vi "Set Or Get Selection Area.vi"(8 "error in (no error)":errorcluster caption="错误输入（无错误）", 9 "Mode":T3, 10 "选择区域输入":T1, 11 "Table Ref In":refnum<vi>) -> (0 "error out":errorcluster caption="错误输出", 2 "选择区域输出":T1, 3 "Table Ref Out":refnum<vi>)   [LabVIEW 2012, in "Table Tool.lvlib"]
uses:
  Table Tool.lvlib
  GetOrSet.ctl
  Selection Area.ctl
  <vilib>/Utility/miscctls.llb/LVRowAndColumnTypeDef.ctl
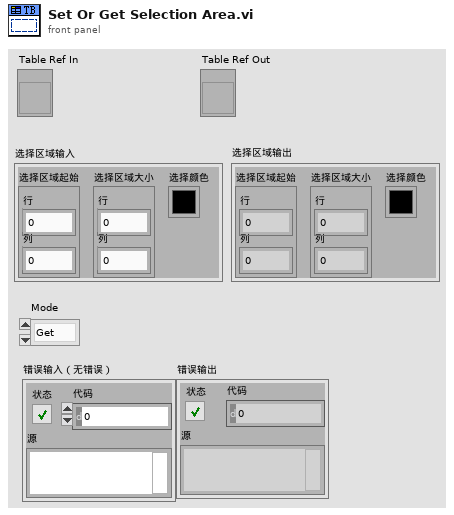
[diagram p1: front panel]
types:
  T1 = typedef "Table Tool.lvlib/Selection Area.ctl" = cluster{"选择区域起始":T2, "选择区域大小":T2, "选择颜色":u32}
  T2 = typedef "LVRowAndColumnTypeDef.ctl" = cluster{"Row":i32, "Column":i32}
  T3 = typedef "Table Tool.lvlib/GetOrSet.ctl" = enum16{"Get", "Set"}
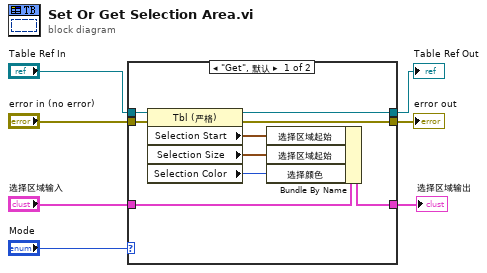
[diagram p0: block diagram]
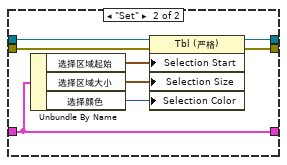
[diagram p2: hidden frame]
diagram:
  n1 = case shown="\"Get\", 默认" "Mode" {
    tunnel: "Table Ref In" -> [w15 w24]
    tunnel: "error in (no error)" -> [w16 w23]
    tunnel: [w13 w22] -> w4
    tunnel: [w14 w21] -> w3
    tunnel: "选择区域输入" -> [w9 w17]
    tunnel: [w8 w17] -> w1
    frame "Get", Default {
      n2 = property class="Tbl (严格)"(reference=w15, error in=w16) -> (reference out=w14:refnum<vi>, error out=w13:errorcluster, "Selection Start"=w12:T2, "Selection Size"=w11:T2, "Selection Color"=w10:u32)
      n3 = Bundle By Name(cluster=w9, "选择区域起始"=w12, "选择区域起始"=w11, "选择颜色"=w10) -> (w8:T1)
    }
    frame "Set" {
      n4 = Unbundle By Name(w17) -> ("选择区域起始"=w20:T2, "选择区域大小"=w19:T2, "选择颜色"=w18:u32)
      n5 = property class="Tbl (严格)"(reference=w24, error in=w23, "Selection Start"=w20, "Selection Size"=w19, "Selection Color"=w18) -> (reference out=w21:refnum<vi>, error out=w22:errorcluster)
    }
  }
  "Table Ref Out" <- w3
  "error out" <- w4
  "选择区域输出" <- w1
